vi "Random Disturbance.vi"(8 "error in (no error)":errorcluster, 11 "Data in":T1={"link 1 angle"=0.0, "link 2 angle"=0.0, "link 1 length"=0.0, "link 2 length"=0.0, "Current arm location"=[{"X"=0.0, "Y"=0.0}, {"X"=-37.249783598972314, "Y"=33.353464914904016}, {"X"=-74.49956719794463, "Y"=66.70692982980803}], "Link Picture"=bytes[1162], "Desired Location"={"Desired X"=0.0, "Desired Y"=0.0}, "Next Location"={"Next X"=0.0, "Next Y"=0.0}, "Error"={"Joint1 error"=0.0, "Joint2 error"=0.0}, "tdms data"=refnum, "de/dt"={"joint1 de/dt"=0.0, "joint2 de/dt"=0.0}, "Voltages"={"Joint1 voltage"=0.0, "Joint2 voltage"=0.0}, "Time"=0.0, "dt"=0.0, "counts/rev"=0.0, "kp"=0.0, "kd"=0.0, "ki"=0.0, "Int(error)"={"joint1 int(e)"=0.0, "joint2 int(e)"=0.0}, "Desired angles"={"theta 1"=0.0, "theta 2"=0.0}, "Current counts"={"theta 1"=0.0, "theta 2"=0.0}, "Desired Counts"={"theta 1"=0.0, "theta 2"=0.0}, "Preivous Error"={"Joint1 Previous error"=0.0, "Joint2 Previous error"=0.0}, "Counts/s"=0.0}) -> (0 "error out":errorcluster, 3 "Data out":T1={"link 1 angle"=0.0, "link 2 angle"=0.0, "link 1 length"=0.0, "link 2 length"=0.0, "Current arm location"=[{"X"=0.0, "Y"=0.0}, {"X"=-37.249783598972314, "Y"=33.353464914904016}, {"X"=-74.49956719794463, "Y"=66.70692982980803}], "Link Picture"=bytes[1162], "Desired Location"={"Desired X"=0.0, "Desired Y"=0.0}, "Next Location"={"Next X"=0.0, "Next Y"=0.0}, "Error"={"Joint1 error"=0.0, "Joint2 error"=0.0}, "tdms data"=refnum, "de/dt"={"joint1 de/dt"=0.0, "joint2 de/dt"=0.0}, "Voltages"={"Joint1 voltage"=0.0, "Joint2 voltage"=0.0}, "Time"=0.0, "dt"=0.0, "counts/rev"=0.0, "kp"=0.0, "kd"=0.0, "ki"=0.0, "Int(error)"={"joint1 int(e)"=0.0, "joint2 int(e)"=0.0}, "Desired angles"={"theta 1"=0.0, "theta 2"=0.0}, "Current counts"={"theta 1"=0.0, "theta 2"=0.0}, "Desired Counts"={"theta 1"=0.0, "theta 2"=0.0}, "Preivous Error"={"Joint1 Previous error"=0.0, "Joint2 Previous error"=0.0}, "Counts/s"=0.0})   [LabVIEW 2016]
uses:
  Type Defs/Host Data.ctl
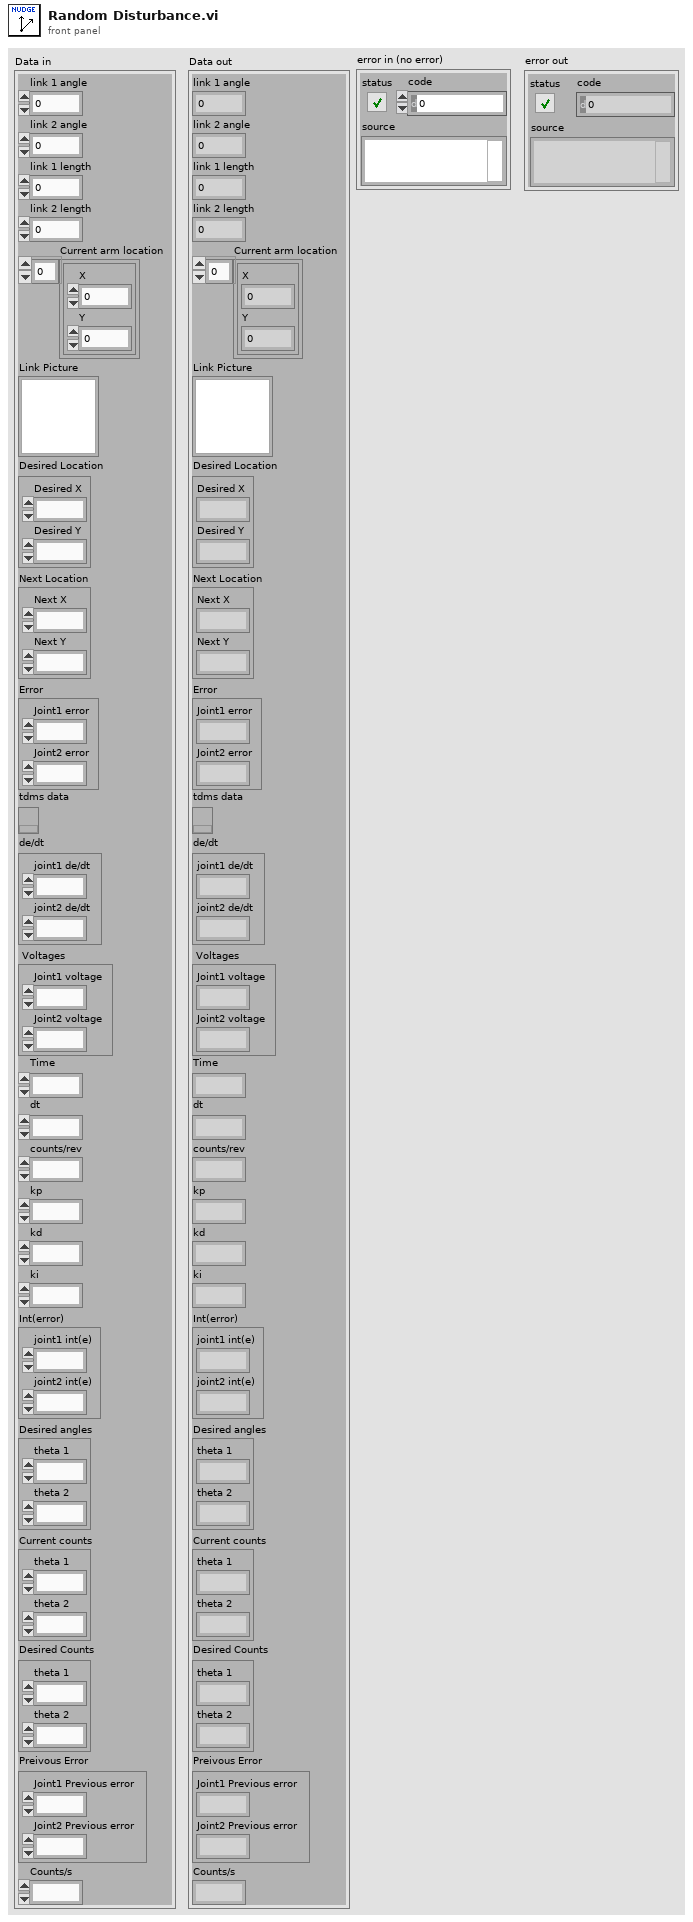
[diagram p1: front panel]
types:
  T1 = typedef "Host Data.ctl" = cluster{"link 1 angle":dbl, "link 2 angle":dbl, "link 1 length":dbl, "link 2 length":dbl, "Current arm location":cluster{"X":dbl, "Y":dbl}[], "Link Picture":picture, "Desired Location":cluster{"Desired X":dbl, "Desired Y":dbl}, "Next Location":cluster{"Next X":dbl, "Next Y":dbl}, "Error":cluster{"Joint1 error":dbl, "Joint2 error":dbl}, "tdms data":refnum<k34>, "de/dt":cluster{"joint1 de/dt":dbl, "joint2 de/dt":dbl}, "Voltages":cluster{"Joint1 voltage":dbl, "Joint2 voltage":dbl}, "Time":dbl, "dt":dbl, "counts/rev":dbl, "kp":dbl, "kd":dbl, "ki":dbl, "Int(error)":cluster{"joint1 int(e)":dbl, "joint2 int(e)":dbl}, "Desired angles":cluster{"theta 1":dbl, "theta 2":dbl}, "Current counts":cluster{"theta 1":dbl, "theta 2":dbl}, "Desired Counts":cluster{"theta 1":dbl, "theta 2":dbl}, "Preivous Error":cluster{"Joint1 Previous error":dbl, "Joint2 Previous error":dbl}, "Counts/s":dbl}
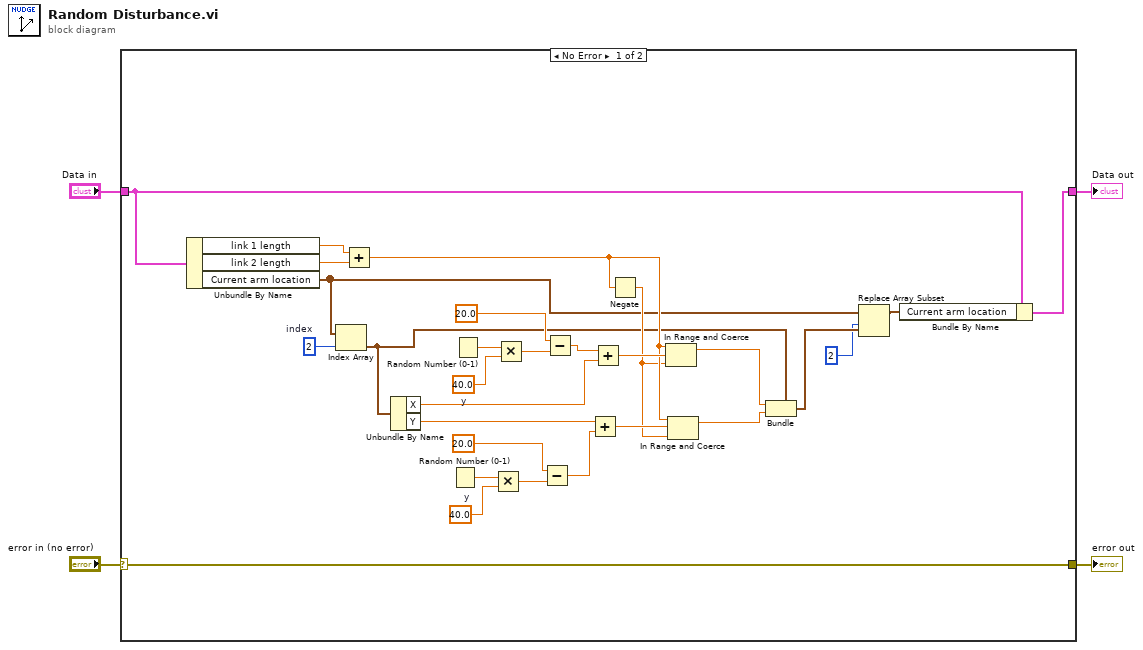
[diagram p0: block diagram]
diagram:
  n1 = case shown="No Error" "error in (no error)" {
    selector: "error in (no error)" -> [w5 w35]
    tunnel: [w5 w35] -> w3
    tunnel: "Data in" -> [w8 w34]
    tunnel: [w7 w34] -> w1
    frame No Error {
      w24 = 40.0  # y
      w31 = 40.0  # y
      w33 = 2  # index
      n2 = Unbundle By Name(w8) -> ("link 1 length"=w18:dbl, "link 2 length"=w17:dbl, "Current arm location"=w11:cluster{"X":dbl, "Y":dbl}[])
      n3 = Index Array(array=w11, index=w33) -> (element=w12:cluster{"X":dbl, "Y":dbl})
      n4 = Add(x=w18, y=w17) -> (x+y=w16:dbl)
      n5 = Unbundle By Name(w12) -> ("X"=w27:dbl, "Y"=w22:dbl)
      n6 = Random Number (0-1)() -> (number: 0 to 1=w23:dbl)
      n7 = Random Number (0-1)() -> (number: 0 to 1=w32:dbl)
      n8 = Multiply(x=w23, y=w24) -> (x*y=w25:dbl)
      n9 = Multiply(x=w32, y=w31) -> (x*y=w30:dbl)
      n10 = Subtract(x=20.0, y=w25) -> (x-y=w21:dbl)
      n11 = Subtract(x=20.0, y=w30) -> (x-y=w28:dbl)
      n12 = Add(x=w22, y=w21) -> (x+y=w19:dbl)
      n13 = Add(x=w28, y=w27) -> (x+y=w20:dbl)
      n14 = Negate(x=w16) -> (-x=w15:dbl)
      n15 = In Range and Coerce(upper limit=w16, x=w20, lower limit=w15) -> (coerced(x)=w14:dbl)  [unwired: 1 out]
      n16 = In Range and Coerce(upper limit=w16, x=w19, lower limit=w15) -> (coerced(x)=w13:dbl)  [unwired: 1 out]
      n17 = Bundle(cluster=w12, "X"=w14, "Y"=w13) -> (w10:cluster{"X":dbl, "Y":dbl})
      n18 = Replace Array Subset(array=w11, new element=w10, index=2) -> (w6:cluster{"X":dbl, "Y":dbl}[])
      n19 = Bundle By Name(cluster=w8, "Current arm location"=w6) -> (w7:T1)
    }
    frame Error {
    }
  }
  "Data out" <- w1
  "error out" <- w3
